vi "test_MixedInstrumentReservation_CallCreateSessions_OnlySpecifiedInstrumentSessionsCreated.vi"(8 "error in":errorcluster) -> (0 "error out":errorcluster, 2 "result":string, 3 "pass":bool)   [LabVIEW 2020, in "MeasurementServerTests.lvlib"]
uses:
  MeasurementServerTests.lvlib
  Helpers/Fake Session Factory/Fake Session Factory.lvclass
  da6ffb6f-c1c9-4957-84dd-e9228483c454.vi
  ffc64c76-1568-41a3-8328-b9126ac9a28d.vi
  Runtime/MeasurementLink Session Management/Session Reservation/Initialize and Close Session Behavior.ctl
  Runtime/MeasurementLink Session Management/Session Reservation/Session Reservation.lvclass
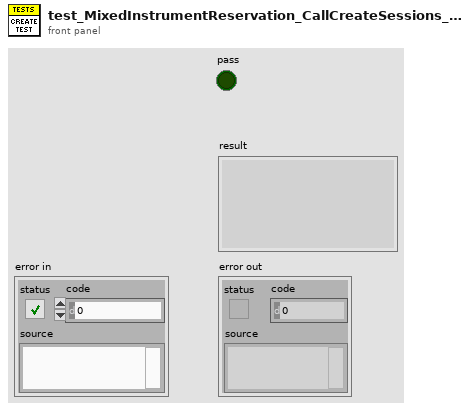
[diagram p1: front panel]
types:
  T1 = typedef "MeasurementLink Session Management.lvlib/Session Reservation.lvclass/Initialize and Close Session Behavior.ctl" = enum16{"Auto", "Initialize and Close", "Attach and Detach", "Initialize and Detach", "Attach and Close"}
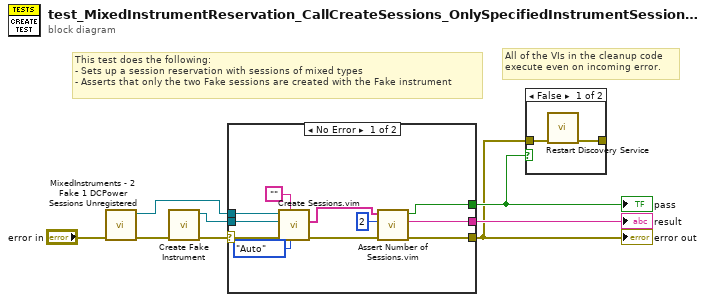
[diagram p0: block diagram]
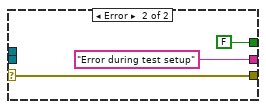
[diagram p2: hidden frame]
diagram:
  # "All of the VIs in the cleanup code\nexecute even on incoming error."
  # "This test does the following:\n- Sets up a session reservation with sessions of mixed types\n- Asserts that only the two Fake sessions are created with the Fake instrument"
  n1 = call "MixedInstruments - 2 Fake 1 DCPower Sessions Unregistered.vi"("error in (no error)"="error in") -> ("error out"=w2:errorcluster, "Session Reservation out"=w1:refnum<class "Session Reservation.lvclass">)  [unwired: 9 in]
  n2 = call "Create Fake Instrument.vi"("error in"=w2) -> ("error out"=w5:errorcluster, "fake instrument out"=w4:refnum<class "Fake Session Factory.lvclass">)  [unwired: 9 in]
  n3 = case shown="No Error" w5 {
    selector: w5 -> [w17 w20]
    tunnel: [w12 w20] -> w6
    tunnel: [w10 FALSE] -> w7
    tunnel: [w11 "Error during test setup" ("f")] -> w8
    tunnel: w4 -> [w19 _]
    tunnel: w1 -> [w18 _]
    frame No Error {
      n4 = call "Create Sessions.vim"("initialize and close session behavior"=Initialize_and_Close_Session_Behavior."Auto", "session type"="", "error in"=w17, "instrument"=w19, "session reservation in"=w18) -> ("error out"=w16:errorcluster, "sessions"=w14:string[])  [unwired: 3 in, 2 out]
      n5 = call "Assert Number of Sessions.vim"("error in"=w16, "expected number of sessions"=2, "sessions"=w14) -> ("error out"=w12:errorcluster, "result"=w11:string, "pass"=w10:bool)  [unwired: 6 in]
    }
    frame Error {
    }
  }
  "error out" <- w6
  "pass" <- w7
  "result" <- w8
  n6 = case shown="False" w7 {
    tunnel: w6 -> [w24 _]
    tunnel: [w23 _] -> _
    frame False {
      n7 = call "Restart Discovery Service.vi"("error in"=w24) -> ("error out"=w23:errorcluster)  [unwired: 10 in]
    }
    frame True {
    }
  }
